vi "Ballard XML Generator.Open Message.vi"(0 "SDI":i32, 4 "minRate (400)":i32=400, 6 "maxRate (400)":i32=400, 7 "messageBufferIDRef (128)":i32=128, 8 "labelDecimal":i32, 9 "name":string, 10 "id":string, 11 "string in":string) -> (3 "string out":string)   [LabVIEW 2017]
uses:
  <vilib>/Utility/error.llb/whitespace.ctl
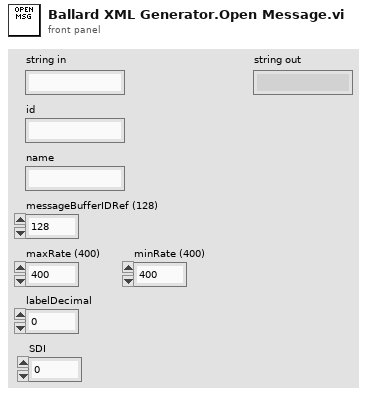
[diagram p1: front panel]
types:
  T1 = typedef "whitespace.ctl" = u16
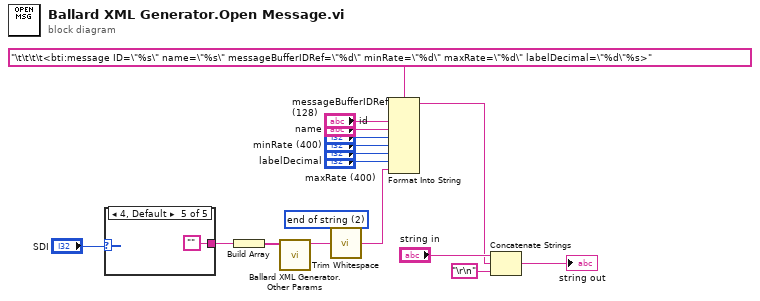
[diagram p0: block diagram]
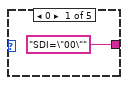
[diagram p2: hidden frame]
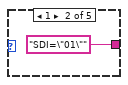
[diagram p3: hidden frame]
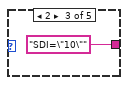
[diagram p4: hidden frame]
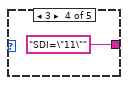
[diagram p5: hidden frame]
diagram:
  w1 = T1 2 items=["both", "start of string", "end of string"] ("location (both)")
  n1 = case shown="4, Default" "SDI" {
    tunnel: ["SDI=\"00\"" "SDI=\"01\"" "SDI=\"10\"" "SDI=\"11\"" ""] -> w5
    frame 0 {
    }
    frame 1 {
    }
    frame 2 {
    }
    frame 3 {
    }
    frame 4, Default {
    }
  }
  n2 = Build Array(w5) -> (w4:string[])
  n3 = call "Ballard XML Generator.Other Params.vi"("other params"=w4) -> ("string"=w3:string)  [unwired: 10 in]
  n4 = call <vilib>:"Trim Whitespace.vi"("string"=w3, "location (both)"=w1) -> ("trimmed string"=w2:string)
  n5 = Format Into String(format string="\t\t\t\t<bti:message ID=\"%s\" name=\"%s\" messageBufferIDRef=\"%d\" minRate=\"%d\" maxRate=\"%d\" labelDecimal=\"%d\"%s>", "id", "name", "messageBufferIDRef (128)", "minRate (400)", "maxRate (400)", "labelDecimal", w2) -> (resulting string=w13:string)  [unwired: 2 in, 1 out]
  n6 = Concatenate Strings("string in", w13, "\r\n") -> (→"string out":string)
